vi "AdjustRanges.vi"(0 "Hardware In":T2 {"Logical Instrument"."Watchdog"."Interval (s)" min=1.0 max=360.0; "Logical Instrument"."Safety Trips"."Pmax Sink Time (s)" min=-1.0; "Logical Instrument"."Safety Trips"."Pmax Sink (W)" min=0.0 format="%#_7g"; "Logical Instrument"."Safety Trips"."Pmax Source Time (s)" min=-1.0; "Logical Instrument"."Safety Trips"."Pmax Source (W)" min=0.0 format="%#_7g"; "Logical Instrument"."Safety Trips"."Absolute Curr Peak" min=0.0; "Logical Instrument"."Safety Trips"."Imax Sink Time (s)" min=-1.0; "Logical Instrument"."Safety Trips"."Imax Sink (A)" min=0.0; "Logical Instrument"."Safety Trips"."Imax Source Time (s)" min=-1.0; "Logical Instrument"."Safety Trips"."Imax Source (A)" min=0.0; "Logical Instrument"."Safety Trips"."Absolute Volt Peak" min=0.0; "Logical Instrument"."Safety Trips"."Vmax Time (s)" min=-1.0; "Logical Instrument"."Safety Trips"."Vmax (V)" min=0.0; "Logical Instrument"."Safety Trips"."Vmin Time (s)" min=-1.0; "Logical Instrument"."Safety Trips"."Vmin (V)" min=0.0; "Logical Instrument"."Aperture (cycles)" min=1 max=64; "Logical Instrument"."FreqOut (Hz)" min=0.0 max=100.0; "Logical Instrument"."Slew Rates"."Phase Angle Min (Deg/s)" min=0.0; "Logical Instrument"."Slew Rates"."Phase Angle Max (Deg/s)" min=0.0; "Logical Instrument"."Slew Rates"."Freq Min (Hz/s)" min=0.0; "Logical Instrument"."Slew Rates"."Freq Max (Hz/s)" min=0.0; "Logical Instrument"."Slew Rates"."Pmax (W/s)" min=0.0; "Logical Instrument"."Slew Rates"."Pmin (W/s)" min=0.0; "Logical Instrument"."Slew Rates"."Imax (A/s)" min=0.0; "Logical Instrument"."Slew Rates"."Vmax (V/s)" min=0.0; "Logical Instrument"."Slew Rates"."Imin (A/s)" min=0.0; "Logical Instrument"."Slew Rates"."Vmin (V/s)" min=0.0; "Logical Instrument"."Phases"."C-Wave Shape" items=["Sine", "User1", "User2", "User3"]; "Logical Instrument"."Phases"."B-Wave Shape" items=["Sine", "User1", "User2", "User3"]; "Logical Instrument"."Phases"."A-Wave Shape" items=["Sine", "User1", "User2", "User3"]; "Logical Instrument"."Phases"."C-Change at..." min=0 max=359; "Logical Instrument"."Phases"."B-Change at..." min=0 max=359; "Logical Instrument"."Phases"."A-Change at..." min=0; "Logical Instrument"."Phases"."C-Angle (Deg)" min=0; "Logical Instrument"."Phases"."B-Angle (Deg)" min=0; "Logical Instrument"."Phases"."C-Volts (V)" min=0.0; "Logical Instrument"."Phases"."B-Volts (V)" min=0.0; "Logical Instrument"."Phases"."A-Volts (V)" min=0.0; "Logical Instrument"."Vout (V)" min=0.0; "Mode" items=["3-Phase AC"=0, "AC"=1, "DC"=2, "AC - AC"=7, "AC - DC"=8, "DC - AC"=11, "DC - DC"=12, "2-Phase AC - AC"=5, "2-Phase AC - DC"=6, "AC - AC - AC"=3, "DC - DC - DC"=4, "AC - AC - DC"=9, "AC - DC - DC"=10, "AC - DC - AC"=13, "DC - AC - AC"=14, "DC - AC - DC"=15]}, 3 "error in (no error)":errorcluster) -> (7 "Hardware Out":T2 {"Logical Instrument"."Watchdog"."Interval (s)" min=1.0 max=360.0; "Logical Instrument"."Safety Trips"."Pmax Sink Time (s)" min=-1.0; "Logical Instrument"."Safety Trips"."Pmax Sink (W)" min=0.0 format="%#_7g"; "Logical Instrument"."Safety Trips"."Pmax Source Time (s)" min=-1.0; "Logical Instrument"."Safety Trips"."Pmax Source (W)" min=0.0 format="%#_7g"; "Logical Instrument"."Safety Trips"."Absolute Curr Peak" min=0.0; "Logical Instrument"."Safety Trips"."Imax Sink Time (s)" min=-1.0; "Logical Instrument"."Safety Trips"."Imax Sink (A)" min=0.0; "Logical Instrument"."Safety Trips"."Imax Source Time (s)" min=-1.0; "Logical Instrument"."Safety Trips"."Imax Source (A)" min=0.0; "Logical Instrument"."Safety Trips"."Absolute Volt Peak" min=0.0; "Logical Instrument"."Safety Trips"."Vmax Time (s)" min=-1.0; "Logical Instrument"."Safety Trips"."Vmax (V)" min=0.0; "Logical Instrument"."Safety Trips"."Vmin Time (s)" min=-1.0; "Logical Instrument"."Safety Trips"."Vmin (V)" min=0.0; "Logical Instrument"."Aperture (cycles)" min=1 max=64; "Logical Instrument"."FreqOut (Hz)" min=0.0 max=100.0; "Logical Instrument"."Slew Rates"."Phase Angle Min (Deg/s)" min=0.0; "Logical Instrument"."Slew Rates"."Phase Angle Max (Deg/s)" min=0.0; "Logical Instrument"."Slew Rates"."Freq Min (Hz/s)" min=0.0; "Logical Instrument"."Slew Rates"."Freq Max (Hz/s)" min=0.0; "Logical Instrument"."Slew Rates"."Pmax (W/s)" min=0.0; "Logical Instrument"."Slew Rates"."Pmin (W/s)" min=0.0; "Logical Instrument"."Slew Rates"."Imax (A/s)" min=0.0; "Logical Instrument"."Slew Rates"."Vmax (V/s)" min=0.0; "Logical Instrument"."Slew Rates"."Imin (A/s)" min=0.0; "Logical Instrument"."Slew Rates"."Vmin (V/s)" min=0.0; "Logical Instrument"."Phases"."C-Wave Shape" items=["Sine", "User1", "User2", "User3"]; "Logical Instrument"."Phases"."B-Wave Shape" items=["Sine", "User1", "User2", "User3"]; "Logical Instrument"."Phases"."A-Wave Shape" items=["Sine", "User1", "User2", "User3"]; "Logical Instrument"."Phases"."C-Change at..." min=0 max=359; "Logical Instrument"."Phases"."B-Change at..." min=0 max=359; "Logical Instrument"."Phases"."A-Change at..." min=0; "Logical Instrument"."Phases"."C-Angle (Deg)" min=0; "Logical Instrument"."Phases"."B-Angle (Deg)" min=0; "Logical Instrument"."Phases"."C-Volts (V)" min=0.0; "Logical Instrument"."Phases"."B-Volts (V)" min=0.0; "Logical Instrument"."Phases"."A-Volts (V)" min=0.0; "Logical Instrument"."Vout (V)" min=0.0; "Mode" items=["3-Phase AC"=0, "AC"=1, "DC"=2, "AC - AC"=7, "AC - DC"=8, "DC - AC"=11, "DC - DC"=12, "2-Phase AC - AC"=5, "2-Phase AC - DC"=6, "AC - AC - AC"=3, "DC - DC - DC"=4, "AC - AC - DC"=9, "AC - DC - DC"=10, "AC - DC - AC"=13, "DC - AC - AC"=14, "DC - AC - DC"=15]}, 10 "error out":errorcluster)   [LabVIEW 2018, in "AcPwrPlugins.lvlib" / "NHRGridSim.lvclass"]
uses:
  NHRGridSim.lvclass
  TypeDefs/NHRGrid_Hardware.ctl
  TypeDefs/NHRGrid_Modes.ctl
  TypeDefs/NHRGrid_Logical_Instrument.ctl
  TypeDefs/NHRGrid_InstrumentCluster.ctl
  TypeDefs/NHRGrid_Phases_Tabs.ctl
  TypeDefs/NHRGrid_SlewRates.ctl
  TypeDefs/NHRGrid_Ranges.ctl
  TypeDefs/NHRGrid_SafetyTrips.ctl
  TypeDefs/NHRGrid_Watchdog.ctl
panel:
  in  "Tab Control":T1(tab)
  # "THIS CAN BE DELETED, WILL NOT BE USED. OLD PRELIM INTERFACE DESIGN"
  # "Degrees with Respect to Phase A"
  # "Voltages (L-N)"
  # "Degrees for Synchronization"
  # "AC Phase Waveform"
  # "Degrees with Respect to Phase A"
  # "Voltages (L-N)"
  # "Degrees for Synchronization"
  # "AC Phase Waveform"
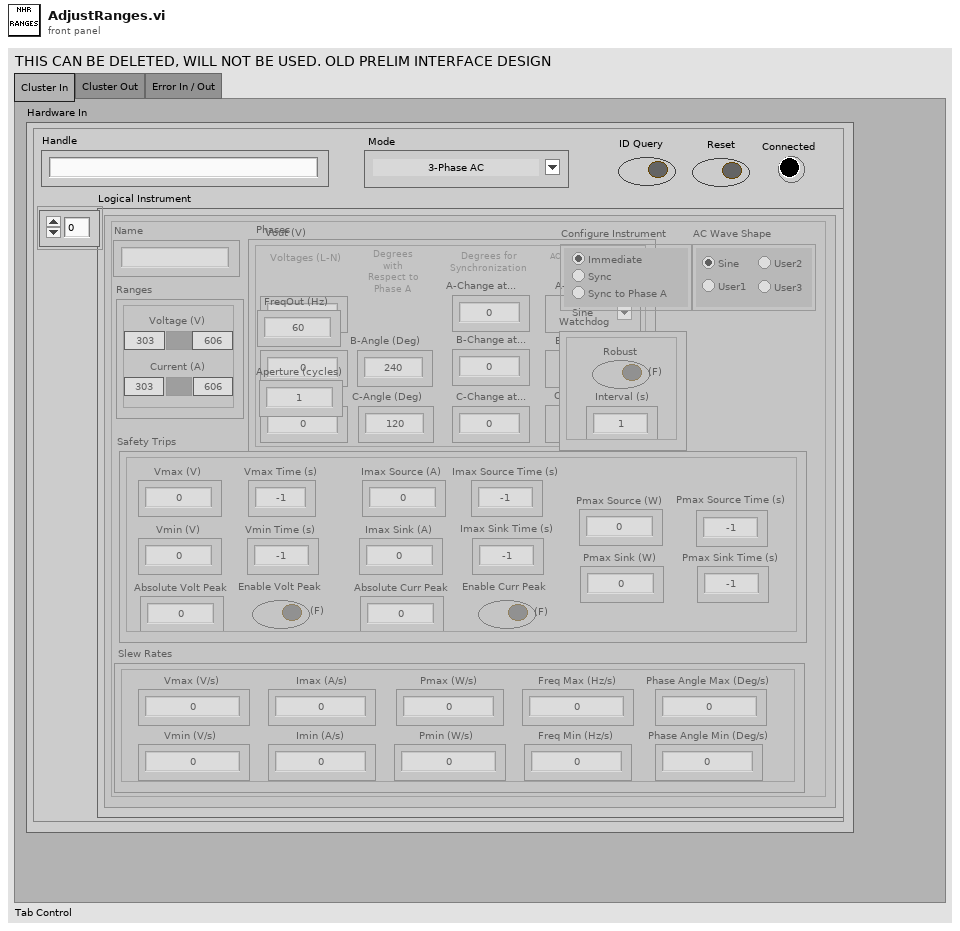
[diagram p1: front panel]
types:
  T1 = enum32{"Cluster In", "Cluster Out", "Error In / Out"}
  T2 = typedef "NHRGrid_Hardware.ctl" = cluster{"Handle":string, "Reset":bool, "Mode":T3, "ID Query":bool, "Connected":bool, "Logical Instrument":T4}
  T3 = typedef "AcPwrPlugins.lvlib/NHRGridSim.lvclass/NHRGrid_Modes.ctl" = u8
  T4 = typedef "AcPwrPlugins.lvlib/NHRGridSim.lvclass/NHRGrid_Logical_Instrument.ctl" = T5[]
  T5 = typedef "AcPwrPlugins.lvlib/NHRGridSim.lvclass/NHRGrid_InstrumentCluster.ctl" = cluster{"Name":string, "Vout (V)":dbl, "VType":string, "Phases":T6, "Slew Rates":T7, "FreqOut (Hz)":dbl, "Aperture (cycles)":i32, "Configure Instrument":enum32{"Conf1", "Conf2", "Conf3"}, "AC Wave Shape":enum32{"Sine", "User1", "User2", "User3"}, "Ranges":T8, "Safety Trips":T9, "Watchdog":T10}
  T6 = typedef "AcPwrPlugins.lvlib/NHRGridSim.lvclass/NHRGrid_Phases_Tabs.ctl" = cluster{"A-Volts (V)":dbl, "B-Volts (V)":dbl, "C-Volts (V)":dbl, "A-Change at...":i32, "B-Angle (Deg)":i32, "C-Angle (Deg)":i32, "B-Change at...":i32, "C-Change at...":i32, "AngleTxt":string, "A-Wave Shape":u16, "B-Wave Shape":u16, "C-Wave Shape":u16}
  T7 = typedef "AcPwrPlugins.lvlib/NHRGridSim.lvclass/NHRGrid_SlewRates.ctl" = cluster{"Vmax (V/s)":dbl, "Vmin (V/s)":dbl, "Imax (A/s)":dbl, "Imin (A/s)":dbl, "Pmax (W/s)":dbl, "Pmin (W/s)":dbl, "Freq Max (Hz/s)":dbl, "Freq Min (Hz/s)":dbl, "Phase Angle Max (Deg/s)":dbl, "Phase Angle Min (Deg/s)":dbl}
  T8 = typedef "AcPwrPlugins.lvlib/NHRGridSim.lvclass/NHRGrid_Ranges.ctl" = cluster{"Voltage (V)":bool, "VHi":dbl, "Current (A)":bool, "CLo":dbl, "CHi":dbl, "VLo":dbl}
  T9 = typedef "AcPwrPlugins.lvlib/NHRGridSim.lvclass/NHRGrid_SafetyTrips.ctl" = cluster{"Vmax (V)":dbl, "Vmin (V)":dbl, "Vmax Time (s)":dbl, "Vmin Time (s)":dbl, "Imax Source (A)":dbl, "Imax Sink (A)":dbl, "Imax Source Time (s)":dbl, "Imax Sink Time (s)":dbl, "Pmax Source (W)":dbl, "Pmax Sink (W)":dbl, "Pmax Source Time (s)":dbl, "Pmax Sink Time (s)":dbl, "Absolute Volt Peak":dbl, "Enable Volt Peak":bool, "Absolute Curr Peak":dbl, "Enable Curr Peak":bool, "Setting t":string, "Recomm t 2":string}
  T10 = typedef "AcPwrPlugins.lvlib/NHRGridSim.lvclass/NHRGrid_Watchdog.ctl" = cluster{"Robust":bool, "Interval (s)":dbl}
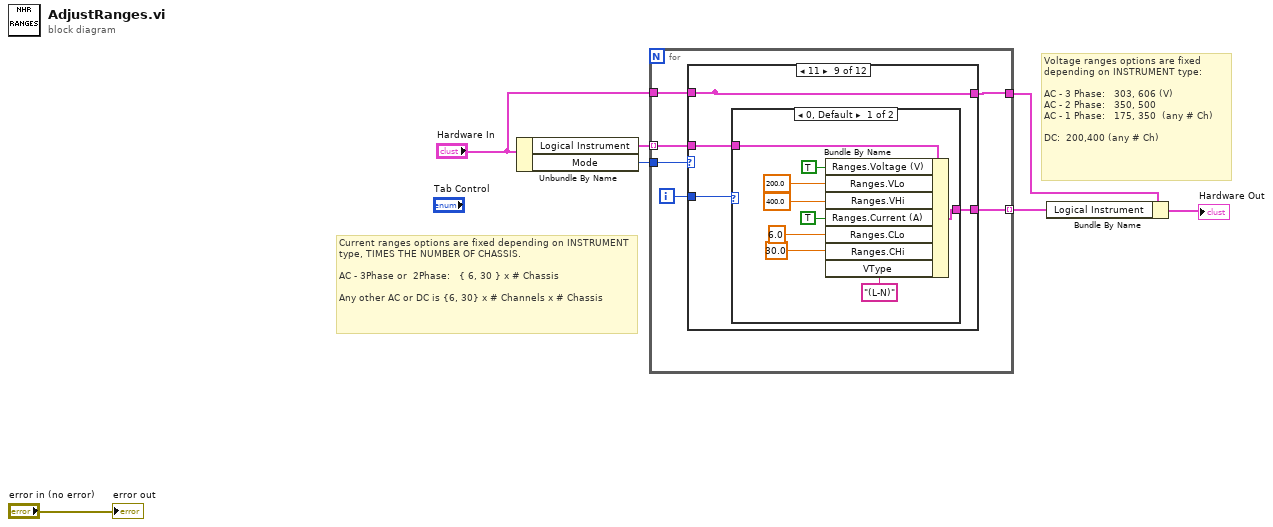
[diagram p0: block diagram]
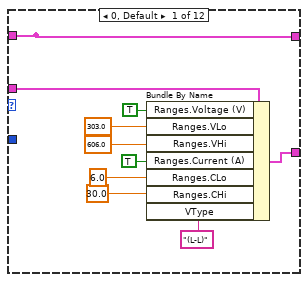
[diagram p2: hidden frame]
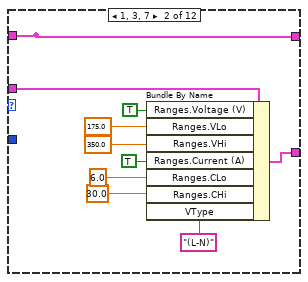
[diagram p3: hidden frame]
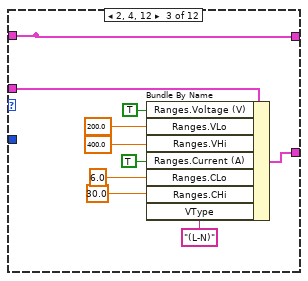
[diagram p4: hidden frame]
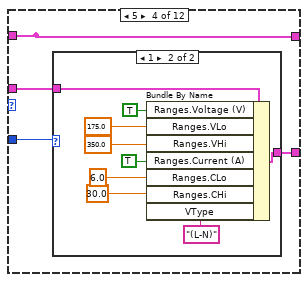
[diagram p5: hidden frame]
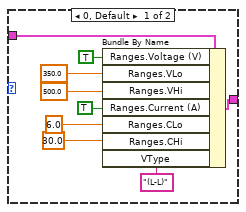
[diagram p6: hidden frame]
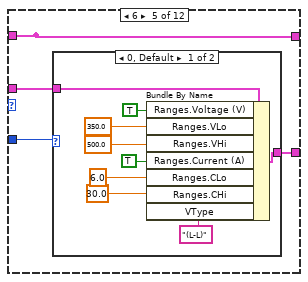
[diagram p7: hidden frame]
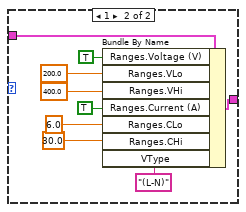
[diagram p8: hidden frame]
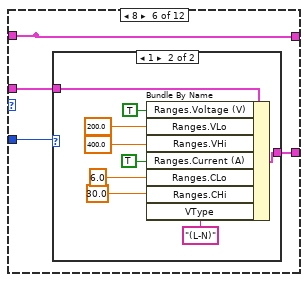
[diagram p9: hidden frame]
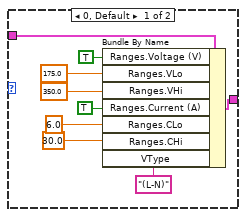
[diagram p10: hidden frame]
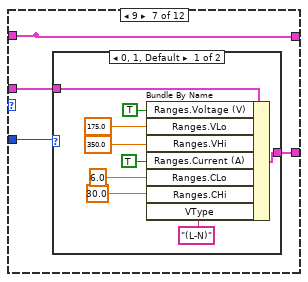
[diagram p11: hidden frame]
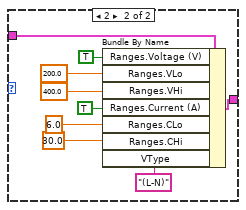
[diagram p12: hidden frame]
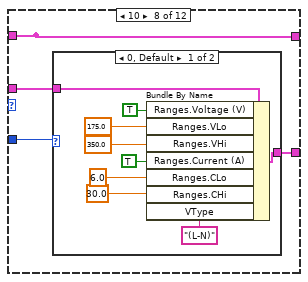
[diagram p13: hidden frame]
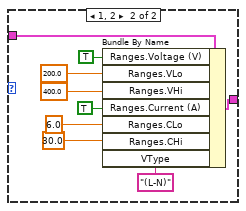
[diagram p14: hidden frame]
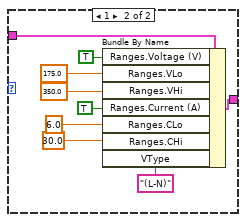
[diagram p15: hidden frame]
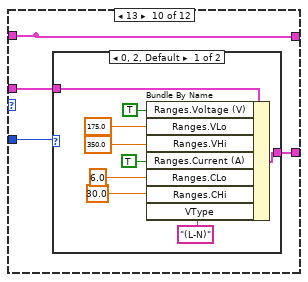
[diagram p16: hidden frame]
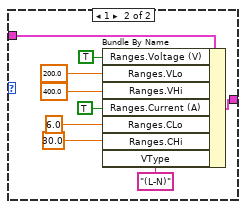
[diagram p17: hidden frame]
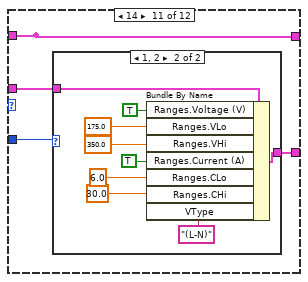
[diagram p18: hidden frame]
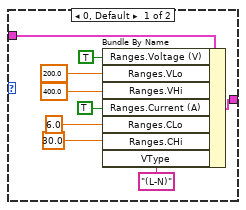
[diagram p19: hidden frame]
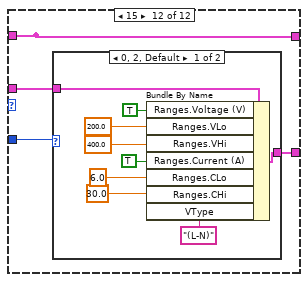
[diagram p20: hidden frame]
diagram:
  # "Current ranges options are fixed depending on INSTRUMENT type, TIMES THE NUMBER OF CHASSIS.\n\nAC - 3Phase or  2Phase:   { 6, 30 } x # Chassis\n\nAny other AC or DC is {6, 30} x # Channels x # Chassis"
  # "Voltage ranges options are fixed \ndepending on INSTRUMENT type:\n\nAC - 3 Phase:   303, 606 (V)\nAC - 2 Phase:   350, 500\nAC - 1 Phase:   175, 350  (any # Ch)\n\nDC:  200,400 (any # Ch)"
  n1 = Unbundle By Name("Hardware In") -> ("Logical Instrument"=w6:T4, "Mode"=w5:T3)
  n2 = for {
    tunnel: w6 -> [w11] mode=indexing
    tunnel: w5 -> [w13]
    tunnel: "Hardware In" -> [w10]
    tunnel: [w9] -> w2
    tunnel: [w8] -> w3 mode=indexing
    i -> [w12]
    n3 = case shown="11" w13 {
      tunnel: w12 -> [_ _ _ w44 w66 w88 w110 w132 w154 w176 w198 w220]
      tunnel: w11 -> [w17 w27 w37 w47 w69 w91 w113 w135 w157 w179 w201 w223]
      tunnel: w10 -> [w16 w26 w36 w46 w68 w90 w112 w134 w156 w178 w200 w222]
      tunnel: [w16 w26 w36 w46 w68 w90 w112 w134 w156 w178 w200 w222] -> _
      tunnel: [w16 w26 w36 w46 w68 w90 w112 w134 w156 w178 w200 w222] -> w9
      tunnel: [w15 w25 w35 w45 w67 w89 w111 w133 w155 w177 w199 w221] -> w8
      frame 0, Default {
        n4 = Bundle By Name(cluster=w17, "Ranges.Voltage (V)"=TRUE ("Ranges.Switch"), "Ranges.VLo"=303.0 ("Ranges.SLo"), "Ranges.VHi"=606.0 ("Ranges.SHi"), "Ranges.Current (A)"=TRUE, "Ranges.CLo"=6.0, "Ranges.CHi"=30.0, "VType"="(L-L)") -> (w15:T5)
      }
      frame 1, 3, 7 {
        n5 = Bundle By Name(cluster=w27, "Ranges.Voltage (V)"=TRUE ("Ranges.Switch"), "Ranges.VLo"=175.0 ("Ranges.SLo"), "Ranges.VHi"=350.0 ("Ranges.SHi"), "Ranges.Current (A)"=TRUE, "Ranges.CLo"=6.0, "Ranges.CHi"=30.0, "VType"="(L-N)") -> (w25:T5)
      }
      frame 2, 4, 12 {
        n6 = Bundle By Name(cluster=w37, "Ranges.Voltage (V)"=TRUE ("Ranges.Switch"), "Ranges.VLo"=200.0 ("Ranges.SLo"), "Ranges.VHi"=400.0 ("Ranges.SHi"), "Ranges.Current (A)"=TRUE, "Ranges.CLo"=6.0, "Ranges.CHi"=30.0, "VType"="(L-N)") -> (w35:T5)
      }
      frame 5 {
        n7 = case shown="1" w44 {
          tunnel: w47 -> [w50 w59]
          tunnel: [w49 w58] -> w45
          frame 0, Default {
            n8 = Bundle By Name(cluster=w50, "Ranges.Voltage (V)"=TRUE ("Ranges.Switch"), "Ranges.VLo"=350.0 ("Ranges.SLo"), "Ranges.VHi"=500.0 ("Ranges.SHi"), "Ranges.Current (A)"=TRUE, "Ranges.CLo"=6.0, "Ranges.CHi"=30.0, "VType"="(L-L)") -> (w49:T5)
          }
          frame 1 {
            n9 = Bundle By Name(cluster=w59, "Ranges.Voltage (V)"=TRUE ("Ranges.Switch"), "Ranges.VLo"=175.0 ("Ranges.SLo"), "Ranges.VHi"=350.0 ("Ranges.SHi"), "Ranges.Current (A)"=TRUE, "Ranges.CLo"=6.0, "Ranges.CHi"=30.0, "VType"="(L-N)") -> (w58:T5)
          }
        }
      }
      frame 6 {
        n10 = case shown="0, Default" w66 {
          tunnel: w69 -> [w72 w81]
          tunnel: [w71 w80] -> w67
          frame 0, Default {
            n11 = Bundle By Name(cluster=w72, "Ranges.Voltage (V)"=TRUE ("Ranges.Switch"), "Ranges.VLo"=350.0 ("Ranges.SLo"), "Ranges.VHi"=500.0 ("Ranges.SHi"), "Ranges.Current (A)"=TRUE, "Ranges.CLo"=6.0, "Ranges.CHi"=30.0, "VType"="(L-L)") -> (w71:T5)
          }
          frame 1 {
            n12 = Bundle By Name(cluster=w81, "Ranges.Voltage (V)"=TRUE ("Ranges.Switch"), "Ranges.VLo"=200.0 ("Ranges.SLo"), "Ranges.VHi"=400.0 ("Ranges.SHi"), "Ranges.Current (A)"=TRUE, "Ranges.CLo"=6.0, "Ranges.CHi"=30.0, "VType"="(L-N)") -> (w80:T5)
          }
        }
      }
      frame 8 {
        n13 = case shown="1" w88 {
          tunnel: w91 -> [w94 w103]
          tunnel: [w93 w102] -> w89
          frame 0, Default {
            n14 = Bundle By Name(cluster=w94, "Ranges.Voltage (V)"=TRUE ("Ranges.Switch"), "Ranges.VLo"=175.0 ("Ranges.SLo"), "Ranges.VHi"=350.0 ("Ranges.SHi"), "Ranges.Current (A)"=TRUE, "Ranges.CLo"=6.0, "Ranges.CHi"=30.0, "VType"="(L-N)") -> (w93:T5)
          }
          frame 1 {
            n15 = Bundle By Name(cluster=w103, "Ranges.Voltage (V)"=TRUE ("Ranges.Switch"), "Ranges.VLo"=200.0 ("Ranges.SLo"), "Ranges.VHi"=400.0 ("Ranges.SHi"), "Ranges.Current (A)"=TRUE, "Ranges.CLo"=6.0, "Ranges.CHi"=30.0, "VType"="(L-N)") -> (w102:T5)
          }
        }
      }
      frame 9 {
        n16 = case shown="0, 1, Default" w110 {
          tunnel: w113 -> [w116 w125]
          tunnel: [w115 w124] -> w111
          frame 0, 1, Default {
            n17 = Bundle By Name(cluster=w116, "Ranges.Voltage (V)"=TRUE ("Ranges.Switch"), "Ranges.VLo"=175.0 ("Ranges.SLo"), "Ranges.VHi"=350.0 ("Ranges.SHi"), "Ranges.Current (A)"=TRUE, "Ranges.CLo"=6.0, "Ranges.CHi"=30.0, "VType"="(L-N)") -> (w115:T5)
          }
          frame 2 {
            n18 = Bundle By Name(cluster=w125, "Ranges.Voltage (V)"=TRUE ("Ranges.Switch"), "Ranges.VLo"=200.0 ("Ranges.SLo"), "Ranges.VHi"=400.0 ("Ranges.SHi"), "Ranges.Current (A)"=TRUE, "Ranges.CLo"=6.0, "Ranges.CHi"=30.0, "VType"="(L-N)") -> (w124:T5)
          }
        }
      }
      frame 10 {
        n19 = case shown="0, Default" w132 {
          tunnel: w135 -> [w138 w147]
          tunnel: [w137 w146] -> w133
          frame 0, Default {
            n20 = Bundle By Name(cluster=w138, "Ranges.Voltage (V)"=TRUE ("Ranges.Switch"), "Ranges.VLo"=175.0 ("Ranges.SLo"), "Ranges.VHi"=350.0 ("Ranges.SHi"), "Ranges.Current (A)"=TRUE, "Ranges.CLo"=6.0, "Ranges.CHi"=30.0, "VType"="(L-N)") -> (w137:T5)
          }
          frame 1, 2 {
            n21 = Bundle By Name(cluster=w147, "Ranges.Voltage (V)"=TRUE ("Ranges.Switch"), "Ranges.VLo"=200.0 ("Ranges.SLo"), "Ranges.VHi"=400.0 ("Ranges.SHi"), "Ranges.Current (A)"=TRUE, "Ranges.CLo"=6.0, "Ranges.CHi"=30.0, "VType"="(L-N)") -> (w146:T5)
          }
        }
      }
      frame 11 {
        n22 = case shown="0, Default" w154 {
          tunnel: w157 -> [w160 w169]
          tunnel: [w159 w168] -> w155
          frame 0, Default {
            n23 = Bundle By Name(cluster=w160, "Ranges.Voltage (V)"=TRUE ("Ranges.Switch"), "Ranges.VLo"=200.0 ("Ranges.SLo"), "Ranges.VHi"=400.0 ("Ranges.SHi"), "Ranges.Current (A)"=TRUE, "Ranges.CLo"=6.0, "Ranges.CHi"=30.0, "VType"="(L-N)") -> (w159:T5)
          }
          frame 1 {
            n24 = Bundle By Name(cluster=w169, "Ranges.Voltage (V)"=TRUE ("Ranges.Switch"), "Ranges.VLo"=175.0 ("Ranges.SLo"), "Ranges.VHi"=350.0 ("Ranges.SHi"), "Ranges.Current (A)"=TRUE, "Ranges.CLo"=6.0, "Ranges.CHi"=30.0, "VType"="(L-N)") -> (w168:T5)
          }
        }
      }
      frame 13 {
        n25 = case shown="0, 2, Default" w176 {
          tunnel: w179 -> [w182 w191]
          tunnel: [w181 w190] -> w177
          frame 0, 2, Default {
            n26 = Bundle By Name(cluster=w182, "Ranges.Voltage (V)"=TRUE ("Ranges.Switch"), "Ranges.VLo"=175.0 ("Ranges.SLo"), "Ranges.VHi"=350.0 ("Ranges.SHi"), "Ranges.Current (A)"=TRUE, "Ranges.CLo"=6.0, "Ranges.CHi"=30.0, "VType"="(L-N)") -> (w181:T5)
          }
          frame 1 {
            n27 = Bundle By Name(cluster=w191, "Ranges.Voltage (V)"=TRUE ("Ranges.Switch"), "Ranges.VLo"=200.0 ("Ranges.SLo"), "Ranges.VHi"=400.0 ("Ranges.SHi"), "Ranges.Current (A)"=TRUE, "Ranges.CLo"=6.0, "Ranges.CHi"=30.0, "VType"="(L-N)") -> (w190:T5)
          }
        }
      }
      frame 14 {
        n28 = case shown="1, 2" w198 {
          tunnel: w201 -> [w204 w213]
          tunnel: [w203 w212] -> w199
          frame 0, Default {
            n29 = Bundle By Name(cluster=w204, "Ranges.Voltage (V)"=TRUE ("Ranges.Switch"), "Ranges.VLo"=200.0 ("Ranges.SLo"), "Ranges.VHi"=400.0 ("Ranges.SHi"), "Ranges.Current (A)"=TRUE, "Ranges.CLo"=6.0, "Ranges.CHi"=30.0, "VType"="(L-N)") -> (w203:T5)
          }
          frame 1, 2 {
            n30 = Bundle By Name(cluster=w213, "Ranges.Voltage (V)"=TRUE ("Ranges.Switch"), "Ranges.VLo"=175.0 ("Ranges.SLo"), "Ranges.VHi"=350.0 ("Ranges.SHi"), "Ranges.Current (A)"=TRUE, "Ranges.CLo"=6.0, "Ranges.CHi"=30.0, "VType"="(L-N)") -> (w212:T5)
          }
        }
      }
      frame 15 {
        n31 = case shown="0, 2, Default" w220 {
          tunnel: w223 -> [w226 w235]
          tunnel: [w225 w234] -> w221
          frame 0, 2, Default {
            n32 = Bundle By Name(cluster=w226, "Ranges.Voltage (V)"=TRUE ("Ranges.Switch"), "Ranges.VLo"=200.0 ("Ranges.SLo"), "Ranges.VHi"=400.0 ("Ranges.SHi"), "Ranges.Current (A)"=TRUE, "Ranges.CLo"=6.0, "Ranges.CHi"=30.0, "VType"="(L-N)") -> (w225:T5)
          }
          frame 1 {
            n33 = Bundle By Name(cluster=w235, "Ranges.Voltage (V)"=TRUE ("Ranges.Switch"), "Ranges.VLo"=175.0 ("Ranges.SLo"), "Ranges.VHi"=350.0 ("Ranges.SHi"), "Ranges.Current (A)"=TRUE, "Ranges.CLo"=6.0, "Ranges.CHi"=30.0, "VType"="(L-N)") -> (w234:T5)
          }
        }
      }
    }
  }
  n34 = Bundle By Name(cluster=w2, "Logical Instrument"=w3) -> (→"Hardware Out":T2)
  "error out" <- "error in (no error)"
